vi "RANGE Analog Calculation.vi"(8 "error in (no error)":errorcluster, 11 "Meter Data":T1={"Meter Size"=0.0, "DAQ Output (Voltage)"=0.0, "Reference (Voltage)"=0.0, "Meter Present"=FALSE, "Meter Visa"="COM3", "Gas Type"="12", "SLPM Error @ Zero"=0.0, "Gas Mix Number"="", "Set STP Register"=FALSE, "Measurement Units"={"Software Rev"="", "Model Number"="", "Manufacturer Info"="", "Software Sub-Rev"="", "Board Rev"="", "Units of Measure Input"={"Abs. Pressure"="", "Gauge/Diff. Press."="", "Barometric Press."="", "Temperature"="", "Volume"="", "Mass"="", "Setpoint"="", "Valve Drive"="", "Totalizer"="", "Tot. Timer"="", "Tot. Avg. Flow"="", "Tot. Peak Flow"=""}}, "Data Frame Format"={"Absolute Pressure"=FALSE, "Gauge/Diff. Pressure"=FALSE, "Barometric Pressure"=FALSE, "Temperature"=FALSE, "Volumetric"=FALSE, "Mass"=FALSE, "Setpoint"=FALSE, "Valve Drive"=FALSE, "Totalizer"=FALSE, "Totalizer Timer"=FALSE, "Totalizer Average Flow"=FALSE, "Totalizer Peak Flow"=FALSE, "Gas Selected"=FALSE, "Tot. Timer Format"=0}}) -> (0 "error out":errorcluster, 2 "Ft³/HR":dbl)   [LabVIEW 2019]
uses:
  Type Definitions/RANGE DAQ Data.ctl
  Drivers/Omega FMA-1600A Series Gas Flow Meter/Type Definitions/FMA1600A Gas Type.ctl
  Drivers/Omega FMA-1600A Series Gas Flow Meter/Type Definitions/FMA1600A Units String.ctl
  Drivers/Alicat Gas Meter Driver/Sub-VIs/Units of Measure.ctl
  Drivers/Alicat Gas Meter Driver/Sub-VIs/Data Frame.ctl
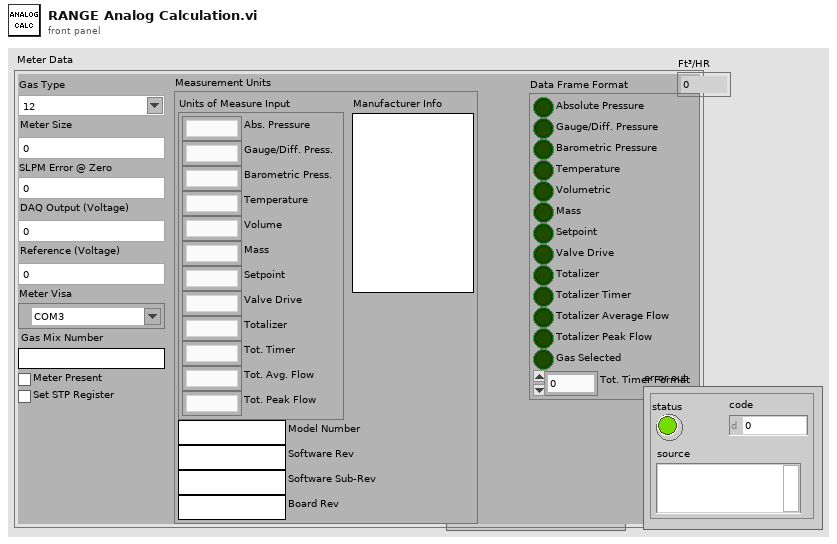
[diagram p1: front panel]
types:
  T1 = typedef "RANGE DAQ Data.ctl" = cluster{"Meter Size":dbl, "DAQ Output (Voltage)":dbl, "Reference (Voltage)":dbl, "Meter Present":bool, "Meter Visa":refnum<visa-resource-name>, "Gas Type":T2, "SLPM Error @ Zero":dbl, "Gas Mix Number":string, "Set STP Register":bool, "Measurement Units":T3, "Data Frame Format":T5}
  T2 = typedef "FMA1600A Gas Type.ctl" = string
  T3 = typedef "FMA1600A Units String.ctl" = cluster{"Software Rev":string, "Model Number":string, "Manufacturer Info":string, "Software Sub-Rev":string, "Board Rev":string, "Units of Measure Input":T4}
  T4 = typedef "Units of Measure.ctl" = cluster{"Abs. Pressure":string, "Gauge/Diff. Press.":string, "Barometric Press.":string, "Temperature":string, "Volume":string, "Mass":string, "Setpoint":string, "Valve Drive":string, "Totalizer":string, "Tot. Timer":string, "Tot. Avg. Flow":string, "Tot. Peak Flow":string}
  T5 = typedef "Data Frame.ctl" = cluster{"Absolute Pressure":bool, "Gauge/Diff. Pressure":bool, "Barometric Pressure":bool, "Temperature":bool, "Volumetric":bool, "Mass":bool, "Setpoint":bool, "Valve Drive":bool, "Totalizer":bool, "Totalizer Timer":bool, "Totalizer Average Flow":bool, "Totalizer Peak Flow":bool, "Gas Selected":bool, "Tot. Timer Format":u16}
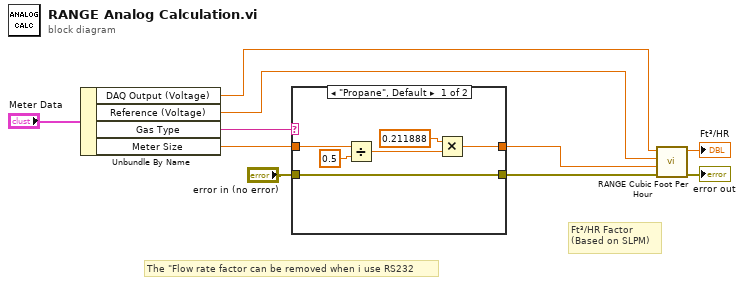
[diagram p0: block diagram]
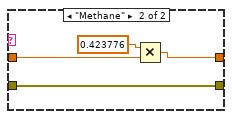
[diagram p2: hidden frame]
diagram:
  # "The \"Flow rate factor can be removed when i use RS232"
  # "Ft³/HR Factor\n(Based on SLPM)"
  n1 = Unbundle By Name("Meter Data") -> ("DAQ Output (Voltage)"=w7:dbl, "Reference (Voltage)"=w8:dbl, "Gas Type"=w2:T2, "Meter Size"=w9:dbl)
  n2 = case shown="\"Propane\", Default" w2 {
    tunnel: [w14 w19] -> w6
    tunnel: w9 -> [w12 w17]
    tunnel: "error in (no error)" -> [w11 w18]
    tunnel: [w11 w18] -> w5
    frame "Propane", Default {
      n3 = Divide(x=w12, y=0.5) -> (x/y=w13:dbl)
      n4 = Multiply(x=0.211888, y=w13) -> (x*y=w14:dbl)
    }
    frame "Methane" {
      n5 = Multiply(x=0.423776, y=w17) -> (x*y=w19:dbl)
    }
  }
  n6 = call "RANGE Cubic Foot Per Hour.vi"("Error In"=w5, "Ft³/HR Factor"=w6, "Reference Voltage"=w8, "DAQ Output (Voltage)"=w7) -> ("Error Out"=→"error out":errorcluster, "Ft³/HR"=→"Ft³/HR":dbl)  [unwired: 6 in]
